vi "Get_Resolved_Path.vi"(8 "error in (no error)":errorcluster, 11 "niLabel in":refnum<class "niLabel.lvclass">) -> (0 "error out":errorcluster, 2 "resolved path":path, 3 "niLabel out":refnum<class "niLabel.lvclass">)   [LabVIEW 2020, in "niLabel.lvclass"]
uses:
  <vilib>/AppBuilder/IB_Classes/Destination/niLabel/niLabel.lvclass
  <vilib>/AppBuilder/IB_Classes/Destination/niLabel/niLabel.lvclass/niLabel.ctl
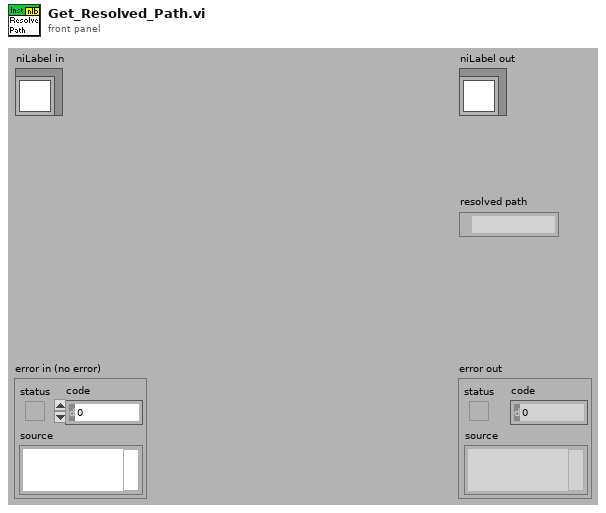
[diagram p1: front panel]
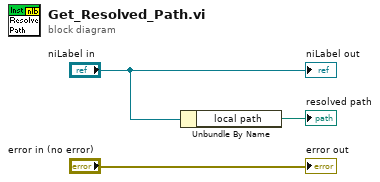
[diagram p0: block diagram]
diagram:
  n1 = Unbundle By Name("niLabel in") -> ("local path"=→"resolved path":path)
  "error out" <- "error in (no error)"
  "niLabel out" <- "niLabel in"
